vi "Keithley 6517 Store and Acquire Trace Data.vi"() -> ()   [LabVIEW 2016]
doc: "This example shows how to store reading to data buffer and then acquire trace data and trace buffer memory usage status.\n\n<B>Note:</B>\nThis Example is ONLY compatible with model 6517."
uses:
  <instrlib>/Keithley 6517/Keithley 6517.lvlib
panel:
  in  "Timeout (10000 ms)":u32=10000
  out "Measurements":T1(array[cluster]) {"Measurement" format="%.6e"}
  in  "Count Value":i32=10
  out "Total Size":i32
  out "Actual Trace Buffer Size":i32=1
  in  "VISA resource name":refnum<visa-resource-name>
  # "(c) 2016-2017 National Instruments.  ALL RIGHTS RESERVED."
  # "Note: This Example is ONLY compatible with model 6517."
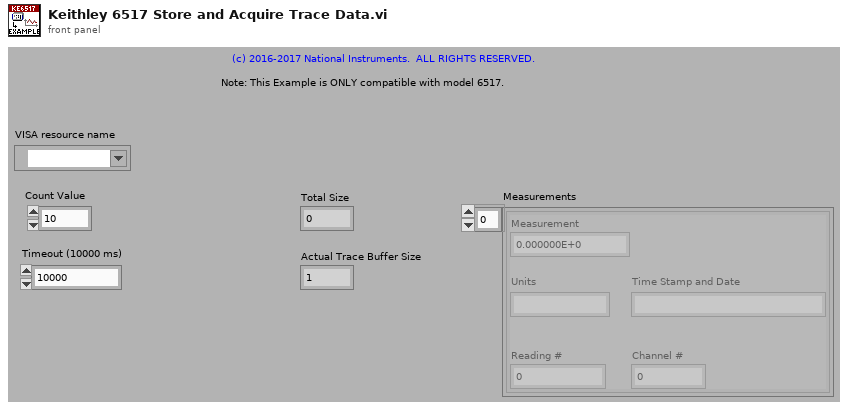
[diagram p1: front panel]
types:
  T1 = cluster{"Measurement":dbl, "Units":string, "Time Stamp and Date":string, "Reading #":dbl, "Channel #":dbl}[]
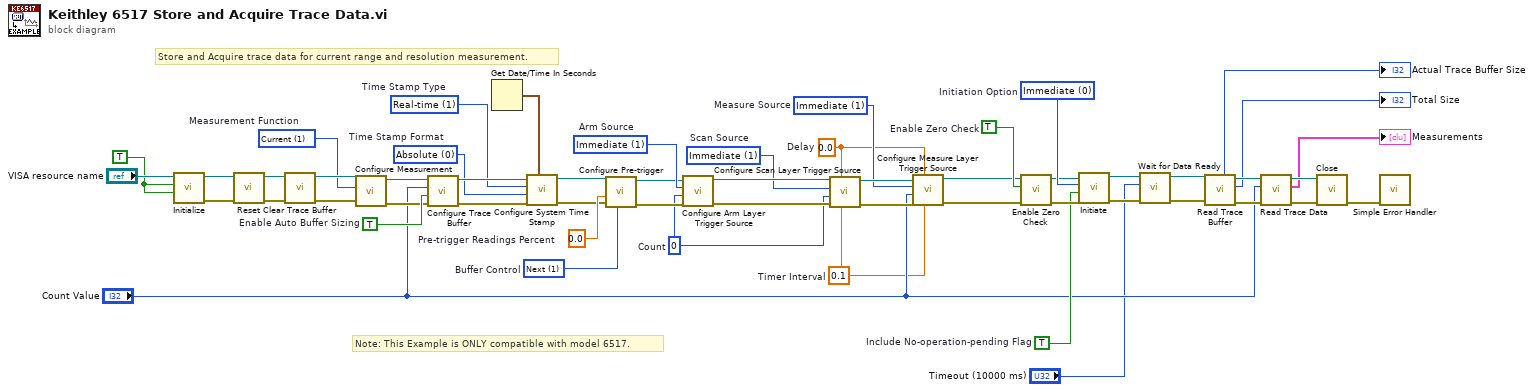
[diagram p0: block diagram]
diagram:
  w9 = 0 items=["Absolute", "Delta"]  # Time Stamp Format
  w10 = 1 items=["Relative-time", "Real-time"]  # Time Stamp Type
  w17 = 0.0  # Pre-trigger Readings Percent
  w18 = 1 items=["Never", "Next", "Always", "Pretrigger"]  # Buffer Control
  w21 = TRUE  # Include No-operation-pending Flag
  w22 = 1 items=["Hold"=0, "Immediate"=1, "Manual"=3, "Bus"=4, "Trigger Link"=5, "External Triggering"=6, "Timer "=7]  # Measure Source
  w6 = 0.1  # Timer Interval
  w7 = 0.0  # Delay
  w23 = 1 items=["Hold"=0, "Immediate"=1, "Manual"=3, "Bus"=4, "Trigger Link"=5, "External Triggering"=6, "Timer "=7]  # Scan Source
  w8 = 0  # Count
  w30 = 1 items=["Hold", "Immediate", "Real-time Clock", "Manual", "Bus", "Trigger Link", "External Triggering"]  # Arm Source
  w31 = 1 items=["Voltage", "Current", "Resistance", "Charge"]  # Measurement Function
  w42 = TRUE  # Enable Zero Check
  w43 = 0 items=["Immediate", "Continuous"]  # Initiation Option
  w47 = TRUE  # Enable Auto Buffer Sizing
  w48 = TRUE ("ID Query (True)")
  # "Note: This Example is ONLY compatible with model 6517."
  # "Store and Acquire trace data for current range and resolution measurement."
  n1 = call <instrlib>:"Initialize.vi"("Reset (True)"=w48, "ID Query (True)"=w48, "VISA resource name"="VISA resource name") -> ("error out"=w37:errorcluster, "VISA resource name out"=w38:refnum<visa-resource-name>)  [unwired: 7 in]
  n2 = call <instrlib>:"Reset.vi"("error in (no error)"=w37, "VISA resource name"=w38) -> ("error out"=w36:errorcluster, "VISA resource name out"=w39:refnum<visa-resource-name>)  [unwired: 8 in]
  n3 = call <instrlib>:"Clear Trace Buffer.vi"("error in (no error)"=w36, "VISA resource name"=w39) -> ("error out"=w33:errorcluster, "VISA resource name out"=w35:refnum<visa-resource-name>)  [unwired: 8 in]
  n4 = call <instrlib>:"Configure Measurement.vi"("error in (no error)"=w33, "Measurement Function (0: Voltage)"=w31, "VISA resource name"=w35) -> ("error out"=w32:errorcluster, "VISA resource name out"=w34:refnum<visa-resource-name>)  [unwired: 7 in]
  n5 = call <instrlib>:"Configure Trace Buffer.vi"("error in (no error)"=w32, "Enable Auto Buffer Sizing (F: Disable)"=w47, "Buffer Size (100)"="Count Value", "VISA resource name"=w34) -> ("error out"=w12:errorcluster, "VISA resource name out"=w14:refnum<visa-resource-name>)  [unwired: 6 in]
  n6 = Get Date/Time In Seconds() -> (seconds since 1Jan1904=w15:timestamp)
  n7 = call <instrlib>:"Configure System Time Stamp.vi"("System Date Time"=w15, "error in (no error)"=w12, "Time Stamp Format (0: Absolute)"=w9, "Time Stamp Type (0: Relative-time)"=w10, "VISA resource name"=w14) -> ("error out"=w11:errorcluster, "VISA resource name out"=w13:refnum<visa-resource-name>)  [unwired: 5 in]
  n8 = call <instrlib>:"Configure Pre-trigger.vi"("Buffer Control (0: Never)"=w18, "error in (no error)"=w11, "Pre-trigger Readings Percent (50)"=w17, "VISA resource name"=w13) -> ("error out"=w19:errorcluster, "VISA resource name out"=w20:refnum<visa-resource-name>)  [unwired: 6 in]
  n9 = call <instrlib>:"Configure Arm Layer Trigger Source.vi"("error in (no error)"=w19, "Arm Count (1)"=w8, "Arm Source (1: Immediate)"=w30, "VISA resource name"=w20) -> ("error out"=w28:errorcluster, "VISA resource name out"=w29:refnum<visa-resource-name>)  [unwired: 6 in]
  n10 = call <instrlib>:"Configure Scan Layer Trigger Source.vi"("Scan Timer Interval (0.1)"=w6, "Scan Delay (0 s)"=w7, "error in (no error)"=w28, "Scan Count (1)"=w8, "Scan Source (1: Immediate)"=w23, "VISA resource name"=w29) -> ("error out"=w24:errorcluster, "VISA resource name out"=w27:refnum<visa-resource-name>)  [unwired: 4 in]
  n11 = call <instrlib>:"Configure Measure Layer Trigger Source.vi"("Measure Timer Interval (0.1)"=w6, "Measure Delay (0 s)"=w7, "error in (no error)"=w24, "Measure Count (1)"="Count Value", "Measure Source (1: Immediate)"=w22, "VISA resource name"=w27) -> ("error out"=w25:errorcluster, "VISA resource name out"=w26:refnum<visa-resource-name>)  [unwired: 4 in]
  n12 = call <instrlib>:"Enable Zero Check.vi"("error in (no error)"=w25, "Enable Zero Check (T: Enable)"=w42, "VISA resource name"=w26) -> ("error out"=w40:errorcluster, "VISA resource name out"=w41:refnum<visa-resource-name>)  [unwired: 7 in]
  n13 = call <instrlib>:"Initiate.vi"("error in (no error)"=w40, "Include No-operation-pending Flag (True)"=w21, "Initiation Option (0: Immediate)"=w43, "VISA resource name"=w41) -> ("error out"=w5:errorcluster, "VISA resource name out"=w4:refnum<visa-resource-name>)  [unwired: 6 in]
  n14 = call <instrlib>:"Wait for Data Ready.vi"("error in (no error)"=w5, "Timeout (10000 ms)"="Timeout (10000 ms)", "VISA resource name"=w4) -> ("error out"=w2:errorcluster, "VISA resource name out"=w3:refnum<visa-resource-name>)  [unwired: 7 in]
  n15 = call <instrlib>:"Read Trace Buffer.vi"("error in (no error)"=w2, "VISA resource name"=w3) -> ("error out"=w54:errorcluster, "Total Size"=→"Total Size":i32, "VISA resource name out"=w53:refnum<visa-resource-name>, "Actual Trace Buffer Size"=→"Actual Trace Buffer Size":i32)  [unwired: 5 in, 1 out]
  n16 = call <instrlib>:"Read Trace Data.vi"("error in (no error)"=w54, "Count Value (1)"="Count Value", "VISA resource name"=w53) -> ("error out"=w50:errorcluster, "Measurements"=→"Measurements":T1, "VISA resource name out"=w51:refnum<visa-resource-name>)  [unwired: 6 in]
  n17 = call <instrlib>:"Close.vi"("error in (no error)"=w50, "VISA resource name"=w51) -> ("error out"=w49:errorcluster)  [unwired: 9 in]
  n18 = call <vilib>:"Simple Error Handler.vi"("error in (no error)"=w49) -> ()  [unwired: 4 in, 5 out]
